vi "Actor Core.vi"(8 "error in":errorcluster, 11 "Nested in":refnum<class "Controls.lvclass">) -> (0 "error out":errorcluster, 3 "Actor out":refnum<class "Actor.lvclass">)   [LabVIEW 2020, in "Controls.lvlib" / "Controls.lvclass"]
doc: "(<B>Filename</B>: Actor Framework.lvlib:Actor.lvclass:Actor Core.vi)\n\nReceives messages to the actor, reacts to them, and initiates any error handling that may shut the actor down.\n\nDescendant classes may override this VI to append parallel tasks for the actor to complete while it handles messages. Overrides use the Call Parent Method node."
uses:
  Controls.lvclass
  <vilib>/ActorFramework/Actor/Actor.lvclass
  <vilib>/ActorFramework/Stop Msg/Stop Msg.lvclass
  C:/Program Files (x86)/National Instruments/LabVIEW 2020/vi.lib/ActorFramework/Actor/Actor.lvclass
  D:/Storage/Source Code/Clase AF/ClaseAF/09 Controls and Indicators AF/Controls/Controls.lvclass
  Business Logic/Business Logic Messages/Update Boolean Msg/Update Boolean Msg.lvclass
  Business Logic/Business Logic Messages/Update Meter Msg/Update Meter Msg.lvclass
panel:
  out "HW ID":dbl
  in  "Boolean":bool
  in  "Knob":dbl(knob) scale=0.0..10.0
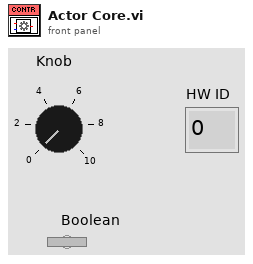
[diagram p1: front panel]
types:
  T1 = cluster{"Stop":refnum<user-event>, "HW ID":refnum<user-event>}
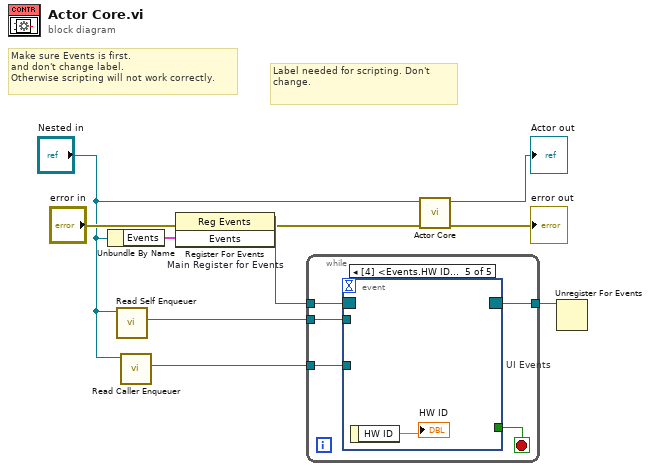
[diagram p0: block diagram]
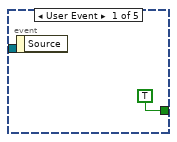
[diagram p2: hidden frame]
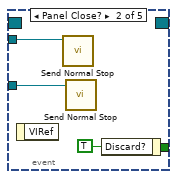
[diagram p3: hidden frame]
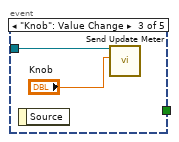
[diagram p4: hidden frame]
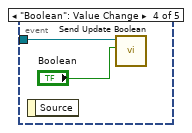
[diagram p5: hidden frame]
diagram:
  # "Label needed for scripting. Don't change."
  # "Make sure Events is first.\nand don't change label.\nOtherwise scripting will not work correctly."
  n1 = Unbundle By Name("Nested in") -> ("Events"=w7:T1)
  n2 = call <vilib>:"Read Self Enqueuer.vi"("Actor"="Nested in") -> ("Self Enqueuer"=w5:refnum<class "Message Enqueuer.lvclass">)  [unwired: 10 in]
  n3 = call <vilib>:"Read Caller Enqueuer.vi"("Actor"="Nested in") -> ("Caller Enqueuer"=w1:refnum<class "Message Enqueuer.lvclass">)  [unwired: 10 in]
  n4 = register-events "Main Register for Events"(error in="error in", w7) -> (reference out=w8:refnum<event-registration>, error out=w3:errorcluster)  [unwired: 1 in]
  n5 = while {
    tunnel: w8 -> [w15]
    tunnel: [w13] -> w6
    tunnel: w5 -> [w12]
    tunnel: w1 -> [w11]
    stop <- w14 stop-if-true
    n6 = event "UI Events" shown="[4] <Events.HW ID>: User Event" {
      selector: w15 -> [_ _ _ _ _]
      dyn-events: [_ _ _ _ _] -> w13
      timeout: _ -> [_ _ _ _ _]
      tunnel: [TRUE _ _ _ _] -> w14
      tunnel: w12 -> [_ w18 _ _ _]
      tunnel: w11 -> [_ w17 w21 w23 _]
      event User Event {
        n7 = event-data() -> ()  [unwired: 1 in, 1 out]
      }
      event Panel Close? {
        n8 = event-data() -> ()  [unwired: 1 in, 1 out]
        n9 = call <vilib>:"Send Normal Stop.vi"("Message Enqueuer"=w18) -> ()  [unwired: 10 in, 1 out]
        n10 = call <vilib>:"Send Normal Stop.vi"("Message Enqueuer"=w17) -> ()  [unwired: 10 in, 1 out]
        n11 = event-data("Discard?"=TRUE) -> ()  [unwired: 1 in, 1 out]
      }
      event "Knob": Value Change {
        n12 = event-data() -> ()  [unwired: 1 in, 1 out]
        n13 = call "Send Update Meter.vi"("Update Meter"="Knob", "Message Enqueuer"=w21) -> ()  [unwired: 8 in, 2 out]
      }
      event "Boolean": Value Change {
        n14 = event-data() -> ()  [unwired: 1 in, 1 out]
        n15 = call "Send Update Boolean.vi"("Boolean"="Boolean", "Message Enqueuer"=w23) -> ()  [unwired: 8 in, 2 out]
      }
      event User Event {
        n16 = event-data() -> ("HW ID"=→"HW ID":dbl)  [unwired: 1 in]
      }
    }
  }
  n17 = call-parent "Actor Core.vi"("error in"=w3, "Actor in"="Nested in") -> ("error out"=→"error out":errorcluster, "Actor out"=→"Actor out":refnum<class "Actor.lvclass">)  [unwired: 8 in]
  n18 = Unregister For Events(event registration refnum=w6) -> ()  [unwired: 1 in, 1 out]
